vi "FTW-Collection-Remove-String.vi"(0 "Collection":refnum<class "FTW-Collection.lvclass">, 5 "Key":string, 7 "Default Value":string, 11 "error in":errorcluster) -> (4 "Collection out":refnum<class "FTW-Collection.lvclass">, 6 "Removed?":bool, 8 "Value":string, 15 "error out":errorcluster)   [LabVIEW 2012, in "FTW-Collection.lvclass"]
uses:
  FTW-Collection.lvclass
  FTW-Collection.lvclass/FTW-Collection.ctl
panel:
  # "Inputs"
  # "Outputs"
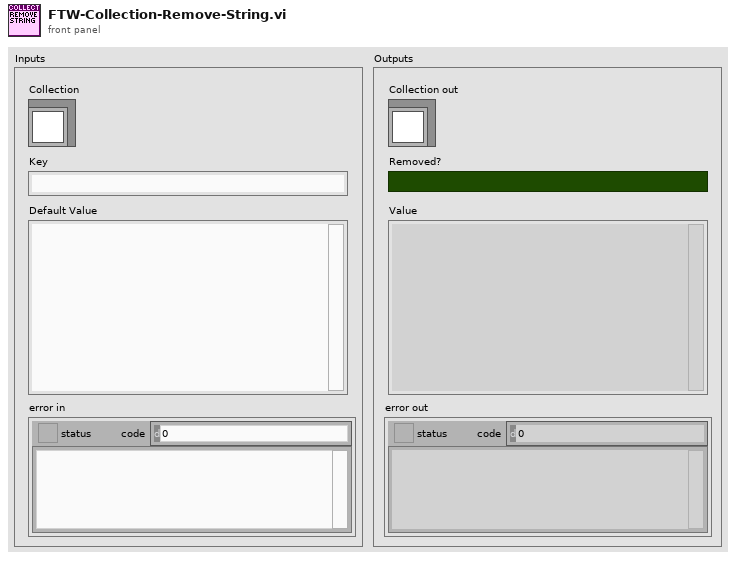
[diagram p1: front panel]
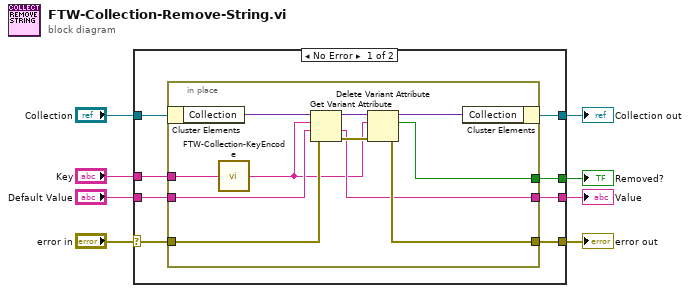
[diagram p0: block diagram]
diagram:
  n1 = case shown="No Error" "error in" {
    selector: "error in" -> [w12 w30]
    tunnel: [w9 w30] -> w8
    tunnel: [w11 _] -> w6
    tunnel: "Collection" -> [w16 w29]
    tunnel: "Key" -> [w14 _]
    tunnel: [w15 w29] -> w3
    tunnel: "Default Value" -> [w13 w28]
    tunnel: [w10 w28] -> w1
    frame No Error {
      n2 = in-place {
        in-place-border: w14 -> [w18]
        in-place-border: [w26] -> w9
        in-place-border: [w25] -> w11
        in-place-border: w13 -> [w24]
        in-place-border: w12 -> [w20]
        in-place-border: [w19] -> w10
        n3 = in-place-cluster #1(w16) -> ("Collection"=w23:variant)
        n4 = call "FTW-Collection-KeyEncode.vi"("Key"=w18) -> ("Encoded Key"=w17:string)
        n5 = Get Variant Attribute(Variant=w23, name=w17, default value (empty Variant)=w24, error in=w20) -> (duplicate Variant=w22:variant, value=w19:string, error out=w21:errorcluster)  [unwired: 1 out]
        n6 = Delete Variant Attribute(4:w21, 6:w17, 7:w22) -> (0:w26:errorcluster, 2:w25:bool, 3:w27:variant)
        n7 = in-place-cluster #1("Collection"=w27) -> (w15:refnum<class "FTW-Collection.lvclass">)
      }
    }
    frame Error {
    }
  }
  "error out" <- w8
  "Removed?" <- w6
  "Collection out" <- w3
  "Value" <- w1
